vi "2dlev-mar xx.vi"(1 "W":dbl[](array[numeric]) format="%.2f", 3 "error":i32, 4 "Coefficients":dbl[](array[numeric]) format="%.2f", 5 "Y":dbl[](array[numeric]) format="%.2f", 6 "X":dbl[](array[numeric]) format="%.2f") -> (0 "chiSqr":dbl format="%.2f")   [LabVIEW 2009]
panel:
  # "Lev-Mar\nXX"
  # "Christian Altenbach\nCaltenba@ucla.edu"
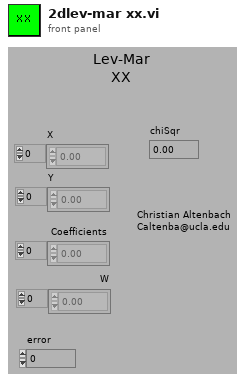
[diagram p1: front panel]
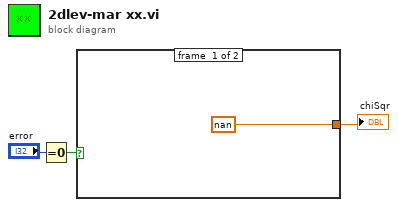
[diagram p0: block diagram]
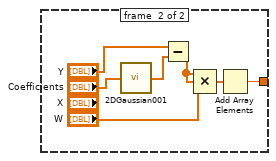
[diagram p2: hidden frame]
diagram:
  n1 = Equal To 0?(x="error") -> (x = 0?=w2:bool)
  n2 = case shown="True" w2 {
    tunnel: [nan w9] -> w1
    frame #0 {
    }
    frame #1 {
      n3 = call "2DGaussian001.vi"("Paramters"="Coefficients") -> ("Flattened Image"=w5:dbl[])
      n4 = Subtract(x="Y", y=w5) -> (x-y=w10:dbl[])
      n5 = Compound Arithmetic op=MULTIPLY(w10, w10, "W") -> (w8:dbl[])
      n6 = Add Array Elements(numeric array=w8) -> (sum=w9:dbl)
    }
  }
  "chiSqr" <- w1
